vi "Panel-OIM.vi"() -> ()   [LabVIEW 2009]
uses:
  Instruments/Motor/Controls/MotorStatus.ctl
  Instruments/Source/Controls/SourceStatus.ctl
panel:
  out "PI2-SourceStatus":T1
  out "PI2-SHUTTER":T2
  out "PI2-CUBE":T2
  out "PI2-LUNETTE":T2
  out "PI2-FI-Z":T2
  out "PI2-FI-Y":T2
  out "PI2-FI-X":T2
  out "PI2-M2-PHI":T2
  out "PI2-M2-THETA":T2
  out "PI2-M1-PHI":T2
  out "PI2-M1-THETA":T2
  out "PI2-P1-Z":T2
  out "PI2-P1-PHI":T2
  out "PI2-P1-THETA":T2
  in  "stop":bool
  out "PI1-SourceStatus":T1
  out "PI1-SHUTTER":T2
  out "PI1-CUBE":T2
  out "PI1-LUNETTE":T2
  out "PI1-FI-Z":T2
  out "PI1-FI-Y":T2
  out "PI1-FI-X":T2
  out "PI1-M2-PHI":T2
  out "PI1-M2-THETA":T2
  out "PI1-M1-PHI":T2
  out "PI1-M1-THETA":T2
  out "PI1-P1-Z":T2
  out "PI1-P1-PHI":T2
  out "PI1-P1-THETA":T2
  # "P1"
  # "P1"
  # "1"
  # "2"
  # "M1"
  # "LUNETTE"
  # "M1"
  # "LUNETTE"
  # "CUBE"
  # "CUBE"
  # "M2"
  # "M2"
  # "SHUTTER"
  # "SHUTTER"
  # "FI"
  # "FI"
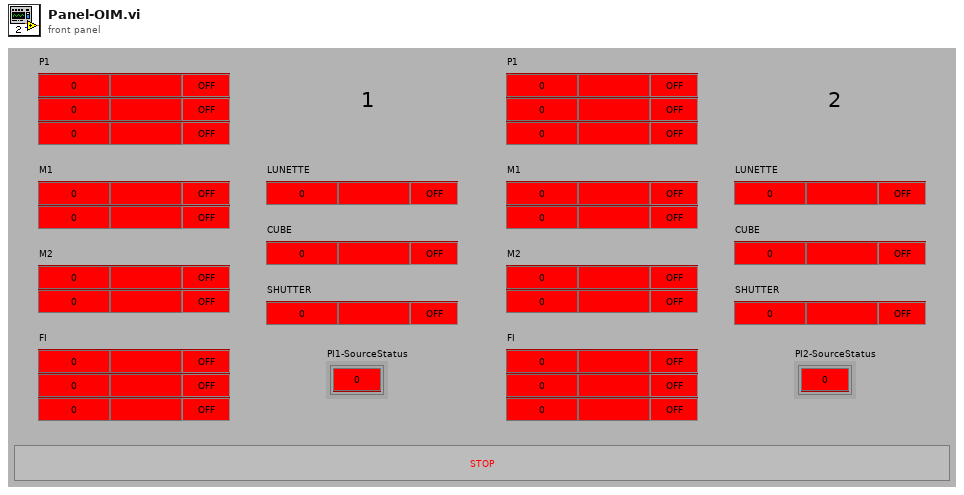
[diagram p1: front panel]
types:
  T1 = typedef "SourceStatus.ctl" = cluster{"Managed?":bool, "Intensity":i32}
  T2 = typedef "MotorStatus.ctl" = cluster{"Managed?":bool, "Position":i32, "Name":string, "Status":enum16{"OFF", "IDLE", "MOVING", "HOMING"}}
  T3 = enum32{"Invalid", "Standard", "Closed", "Hidden", "Minimized", "Maximized"}
  T4 = enum32{"Bad", "Idle", "Run top level", "Running"}
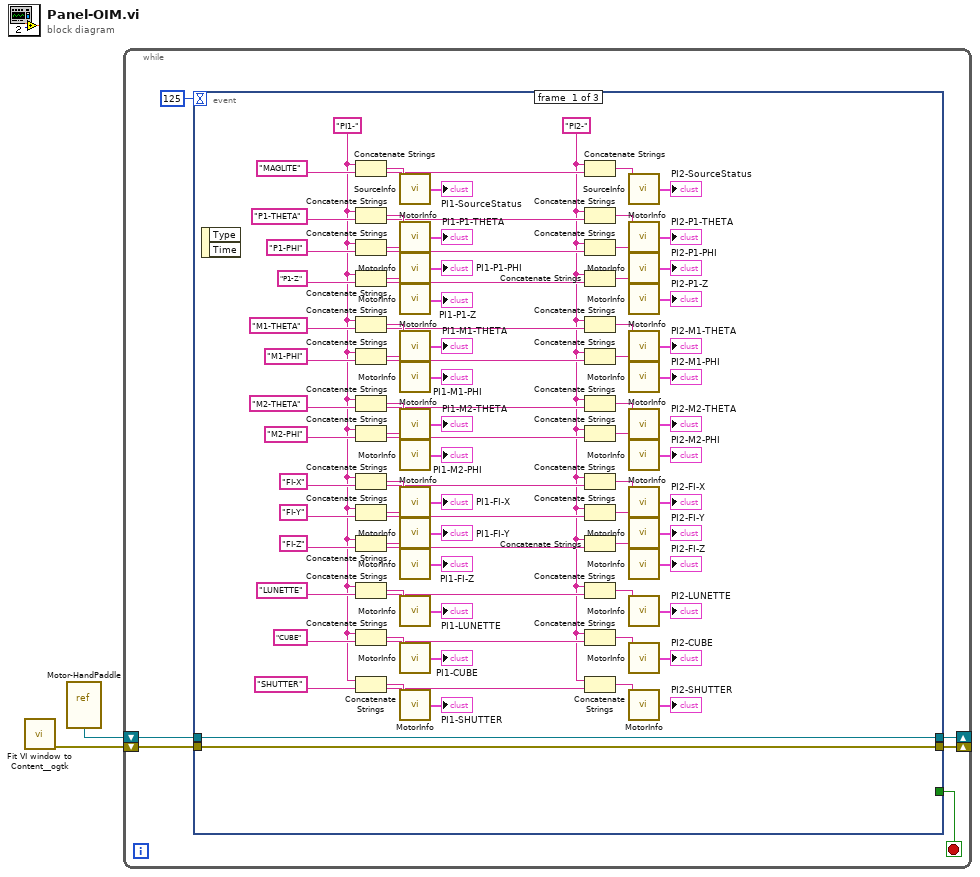
[diagram p0: block diagram]
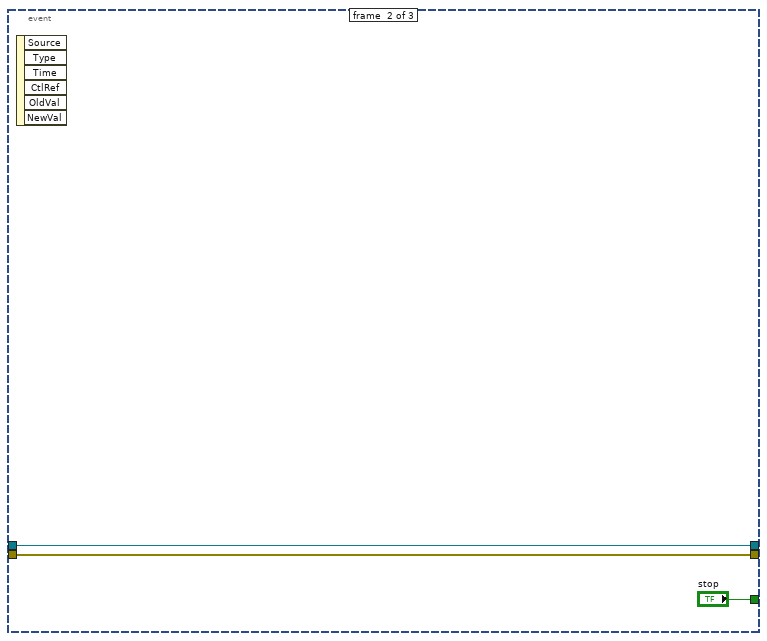
[diagram p2: hidden frame]
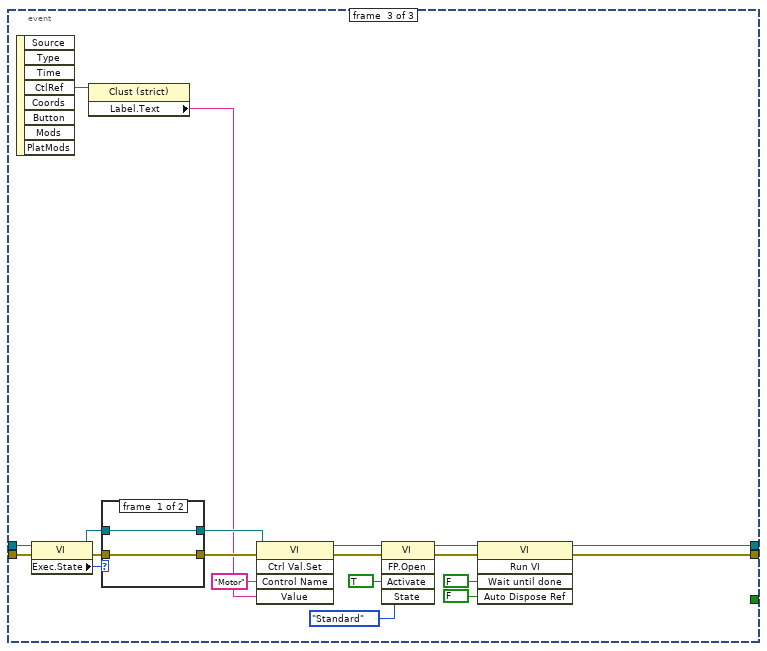
[diagram p3: hidden frame]
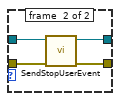
[diagram p4: hidden frame]
diagram:
  n1 = call <userlib>:"Fit VI window to Content__ogtk.vi"() -> ("error out"=w2:errorcluster)  [unwired: 3 in, 4 out]
  n2 = vi-ref "Motor-HandPaddle.vi"() -> (w1:refnum<vi>)
  n3 = while {
    shift-right: [w5] -> _
    shift-left: w2 -> [w6]
    shift-right: [w3] -> _
    shift-left: w1 -> [w4]
    stop <- w7 stop-if-true
    n4 = event shown="[2] \"PI1-P1-THETA\", \"PI1-P1-PHI\", \"PI1-P1-Z\", \"PI1-M1-THETA\", \"PI1-M1-PHI\", \"PI1-M2-THETA\", \"PI1-M2-PHI\", \"PI1-FI-X\", \"PI1-FI-Y\", \"PI1-FI-Z\", \"PI1-LUNETTE\", \"PI1-CUBE\", \"PI1-SHUTTER\", \"PI2-P1-THETA\", \"PI2-P1-PHI\", \"PI2-P1-Z\", \"PI2-M1-THETA\", \"PI2-M1-PHI\", \"PI2-M2-THETA\", \"PI2-M2-PHI\", \"PI2-FI-X\", \"PI2-FI-Y\", \"PI2-FI-Z\", \"PI2-LUNETTE\", \"PI2-CUBE\", \"PI2-SHUTTER\": Mouse Down" {
      selector: _ -> [_ _ _]
      dyn-events: _ -> [_ _ _]
      timeout: 125 -> [_ _ _]
      tunnel: [_ "stop" _] -> w7
      tunnel: w6 -> [w68 w84 w90]
      tunnel: [w68 w84 w89] -> w5
      tunnel: w4 -> [w67 w83 w88]
      tunnel: [w67 w83 w87] -> w3
      event #0 {
        w9 = "PI2-"
        w10 = "PI1-"
        w24 = "MAGLITE" ("Source")
        w11 = "SHUTTER" ("Motor")
        w12 = "CUBE" ("Motor")
        w13 = "LUNETTE" ("Motor")
        w14 = "FI-Z" ("Motor")
        w15 = "FI-Y" ("Motor")
        w16 = "FI-X" ("Motor")
        w17 = "M2-PHI" ("Motor")
        w18 = "M2-THETA" ("Motor")
        w19 = "M1-PHI" ("Motor")
        w20 = "M1-THETA" ("Motor")
        w21 = "P1-Z" ("Motor")
        w22 = "P1-PHI" ("Motor")
        w23 = "P1-THETA" ("Motor")
        n5 = event-data() -> ()  [unwired: 3 out]
        n6 = Concatenate Strings(w10, w24) -> (w66:string)
        n7 = Concatenate Strings(w10, w23) -> (w53:string)
        n8 = Concatenate Strings(w10, w22) -> (w54:string)
        n9 = Concatenate Strings(w10, w21) -> (w55:string)
        n10 = Concatenate Strings(w10, w20) -> (w57:string)
        n11 = Concatenate Strings(w10, w19) -> (w56:string)
        n12 = Concatenate Strings(w10, w18) -> (w61:string)
        n13 = Concatenate Strings(w10, w17) -> (w62:string)
        n14 = Concatenate Strings(w10, w16) -> (w60:string)
        n15 = Concatenate Strings(w10, w15) -> (w59:string)
        n16 = Concatenate Strings(w10, w14) -> (w58:string)
        n17 = Concatenate Strings(w10, w13) -> (w63:string)
        n18 = Concatenate Strings(w10, w12) -> (w64:string)
        n19 = Concatenate Strings(w10, w11) -> (w65:string)
        n20 = call "SourceInfo.vi"("Source"=w66) -> ("SourceStatus"=→"PI1-SourceStatus":T1)  [unwired: 1 in, 7 out]
        n21 = call "MotorInfo.vi"("Motor"=w53) -> ("Axis status"=→"PI1-P1-THETA":T2)  [unwired: 1 in, 7 out]
        n22 = call "MotorInfo.vi"("Motor"=w54) -> ("Axis status"=→"PI1-P1-PHI":T2)  [unwired: 1 in, 7 out]
        n23 = call "MotorInfo.vi"("Motor"=w55) -> ("Axis status"=→"PI1-P1-Z":T2)  [unwired: 1 in, 7 out]
        n24 = call "MotorInfo.vi"("Motor"=w57) -> ("Axis status"=→"PI1-M1-THETA":T2)  [unwired: 1 in, 7 out]
        n25 = call "MotorInfo.vi"("Motor"=w56) -> ("Axis status"=→"PI1-M1-PHI":T2)  [unwired: 1 in, 7 out]
        n26 = call "MotorInfo.vi"("Motor"=w61) -> ("Axis status"=→"PI1-M2-THETA":T2)  [unwired: 1 in, 7 out]
        n27 = call "MotorInfo.vi"("Motor"=w62) -> ("Axis status"=→"PI1-M2-PHI":T2)  [unwired: 1 in, 7 out]
        n28 = call "MotorInfo.vi"("Motor"=w60) -> ("Axis status"=→"PI1-FI-X":T2)  [unwired: 1 in, 7 out]
        n29 = call "MotorInfo.vi"("Motor"=w59) -> ("Axis status"=→"PI1-FI-Y":T2)  [unwired: 1 in, 7 out]
        n30 = call "MotorInfo.vi"("Motor"=w58) -> ("Axis status"=→"PI1-FI-Z":T2)  [unwired: 1 in, 7 out]
        n31 = call "MotorInfo.vi"("Motor"=w63) -> ("Axis status"=→"PI1-LUNETTE":T2)  [unwired: 1 in, 7 out]
        n32 = call "MotorInfo.vi"("Motor"=w64) -> ("Axis status"=→"PI1-CUBE":T2)  [unwired: 1 in, 7 out]
        n33 = call "MotorInfo.vi"("Motor"=w65) -> ("Axis status"=→"PI1-SHUTTER":T2)  [unwired: 1 in, 7 out]
        n34 = Concatenate Strings(w9, w24) -> (w39:string)
        n35 = Concatenate Strings(w9, w23) -> (w52:string)
        n36 = Concatenate Strings(w9, w22) -> (w51:string)
        n37 = Concatenate Strings(w9, w21) -> (w50:string)
        n38 = Concatenate Strings(w9, w20) -> (w48:string)
        n39 = Concatenate Strings(w9, w19) -> (w49:string)
        n40 = Concatenate Strings(w9, w18) -> (w44:string)
        n41 = Concatenate Strings(w9, w17) -> (w43:string)
        n42 = Concatenate Strings(w9, w16) -> (w45:string)
        n43 = Concatenate Strings(w9, w15) -> (w46:string)
        n44 = Concatenate Strings(w9, w14) -> (w47:string)
        n45 = Concatenate Strings(w9, w13) -> (w42:string)
        n46 = Concatenate Strings(w9, w12) -> (w41:string)
        n47 = Concatenate Strings(w9, w11) -> (w40:string)
        n48 = call "SourceInfo.vi"("Source"=w39) -> ("SourceStatus"=→"PI2-SourceStatus":T1)  [unwired: 1 in, 7 out]
        n49 = call "MotorInfo.vi"("Motor"=w52) -> ("Axis status"=→"PI2-P1-THETA":T2)  [unwired: 1 in, 7 out]
        n50 = call "MotorInfo.vi"("Motor"=w51) -> ("Axis status"=→"PI2-P1-PHI":T2)  [unwired: 1 in, 7 out]
        n51 = call "MotorInfo.vi"("Motor"=w50) -> ("Axis status"=→"PI2-P1-Z":T2)  [unwired: 1 in, 7 out]
        n52 = call "MotorInfo.vi"("Motor"=w48) -> ("Axis status"=→"PI2-M1-THETA":T2)  [unwired: 1 in, 7 out]
        n53 = call "MotorInfo.vi"("Motor"=w49) -> ("Axis status"=→"PI2-M1-PHI":T2)  [unwired: 1 in, 7 out]
        n54 = call "MotorInfo.vi"("Motor"=w44) -> ("Axis status"=→"PI2-M2-THETA":T2)  [unwired: 1 in, 7 out]
        n55 = call "MotorInfo.vi"("Motor"=w43) -> ("Axis status"=→"PI2-M2-PHI":T2)  [unwired: 1 in, 7 out]
        n56 = call "MotorInfo.vi"("Motor"=w45) -> ("Axis status"=→"PI2-FI-X":T2)  [unwired: 1 in, 7 out]
        n57 = call "MotorInfo.vi"("Motor"=w46) -> ("Axis status"=→"PI2-FI-Y":T2)  [unwired: 1 in, 7 out]
        n58 = call "MotorInfo.vi"("Motor"=w47) -> ("Axis status"=→"PI2-FI-Z":T2)  [unwired: 1 in, 7 out]
        n59 = call "MotorInfo.vi"("Motor"=w42) -> ("Axis status"=→"PI2-LUNETTE":T2)  [unwired: 1 in, 7 out]
        n60 = call "MotorInfo.vi"("Motor"=w41) -> ("Axis status"=→"PI2-CUBE":T2)  [unwired: 1 in, 7 out]
        n61 = call "MotorInfo.vi"("Motor"=w40) -> ("Axis status"=→"PI2-SHUTTER":T2)  [unwired: 1 in, 7 out]
      }
      event #1 {
        n62 = event-data() -> ()  [unwired: 7 out]
      }
      event #2 {
        n63 = event-data() -> ("CtlRef"=w91:refnum<vi>)  [unwired: 8 out]
        n64 = property class="VI"(reference=w88, error in=w90) -> (reference out=w93:refnum<vi>, error out=w94:errorcluster, "Exec.State"=w96:T4)
        n65 = property class="Clust (strict)"(reference=w91) -> ("Label.Text"=w86:string)  [unwired: 1 in, 2 out]
        n66 = case shown="\"Run top level\", \"Running\"" w96 {
          tunnel: w93 -> [w107 w111]
          tunnel: [w107 w108] -> w92
          tunnel: [w106 w109] -> w95
          tunnel: w94 -> [w106 w110]
          frame #0 {
          }
          frame #1 {
            n67 = call "SendStopUserEvent.vi"("VI Refnum in"=w111, "error in"=w110) -> ("VI Refnum out"=w108:refnum<vi>, "error out"=w109:errorcluster)  [unwired: 6 out]
          }
        }
        n68 = invoke class="VI" method="Ctrl Val.Set"(reference=w92, error in=w95, "Control Name"="Motor", "Value"=w86) -> (reference out=w97:refnum<vi>, error out=w102:errorcluster)  [unwired: 1 in, 3 out]
        n69 = invoke class="VI" method="FP.Open"(reference=w97, error in=w102, "Activate"=TRUE ("Activate?"), "State"=T3."Standard") -> (reference out=w100:refnum<vi>, error out=w101:errorcluster)  [unwired: 1 in, 3 out]
        n70 = invoke class="VI" method="Run VI"(reference=w100, error in=w101, "Wait until done"=FALSE ("Wait Until Done"), "Auto Dispose Ref"=FALSE ("Auto Dispose Reference")) -> (reference out=w87:refnum<vi>, error out=w89:errorcluster)  [unwired: 1 in, 3 out]
      }
    }
  }
